vi "Set Delay.vi"(0 "VISA resource name":refnum<visa-resource-name>, 7 "Delay":dbl=0.5, 11 "error in (no error)":errorcluster) -> (4 "VISA resource name out":refnum<visa-resource-name>, 15 "error out":errorcluster)   [LabVIEW 2020, in "Associated Research 78XX Series.lvlib"]
doc: "SD <step number>\nDeletes the step indicated by the number from the setup file sequence. All step after this\nstep will move up and be renumbered accordingly."
uses:
  <instrlib>/Associated Research 78XX Series/Associated Research 78XX Series.lvlib
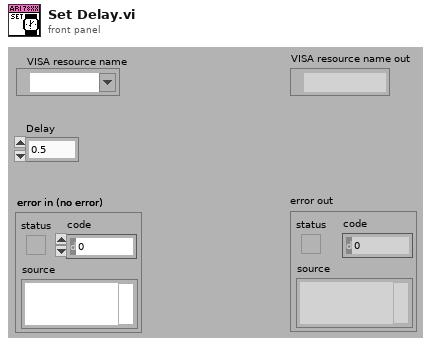
[diagram p1: front panel]
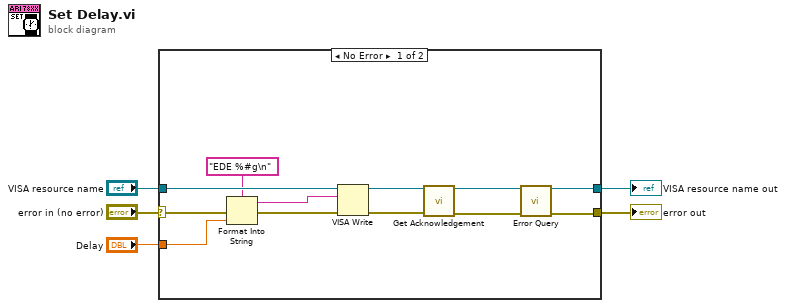
[diagram p0: block diagram]
diagram:
  n1 = case shown="No Error" "error in (no error)" {
    selector: "error in (no error)" -> [w15 w19]
    tunnel: [w14 w19] -> w4
    tunnel: [w16 w18] -> w2
    tunnel: "VISA resource name" -> [w17 w18]
    tunnel: "Delay" -> [w13 _]
    frame No Error {
      n2 = Format Into String(format string="EDE %#g\n" ("\"False\" Command"), error in=w15, w13) -> (resulting string=w8:string, error out=w11:errorcluster)  [unwired: 1 in]
      n3 = VISA Write(VISA resource name=w17, write buffer=w8, error in (no error)=w11) -> (VISA resource name out=w7:refnum<visa-resource-name>, error out=w6:errorcluster)  [unwired: 1 out]
      n4 = call <instrlib>:"Get Acknowledgement.vi"("VISA resource name"=w7, "error in (no error)"=w6) -> ("VISA resource name out"=w10:refnum<visa-resource-name>, "error out"=w9:errorcluster)  [unwired: 12 in]
      n5 = call <instrlib>:"Error Query.vi"("VISA resource name"=w10, "error in (no error)"=w9) -> ("VISA resource name out"=w16:refnum<visa-resource-name>, "error out"=w14:errorcluster)  [unwired: 10 in, 2 out]
    }
    frame Error {
    }
  }
  "error out" <- w4
  "VISA resource name out" <- w2
